vi "grafico2.vi"() -> ()   [LabVIEW 2013]
panel:
  in  "Dial":dbl(knob)
  out "Waveform Chart":dbl(graph)
  out "señal ampl 0,5 a -0,5":dbl(graph)
  in  "Numeric 3":i32
  out "Numeric 2":i32
  out "senal ampl a 5":dbl(graph)
  out "Numeric":dbl
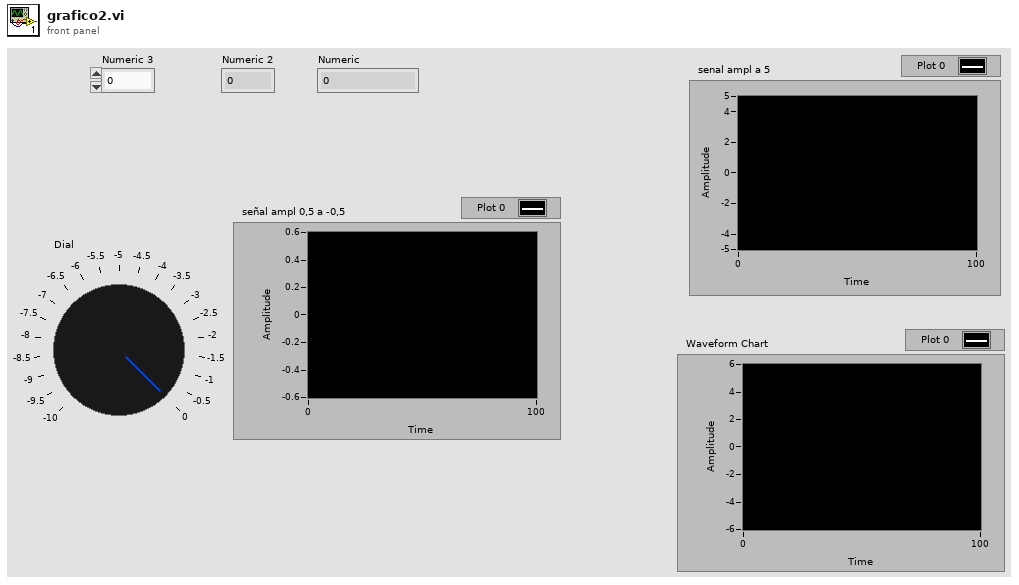
[diagram p1: front panel]
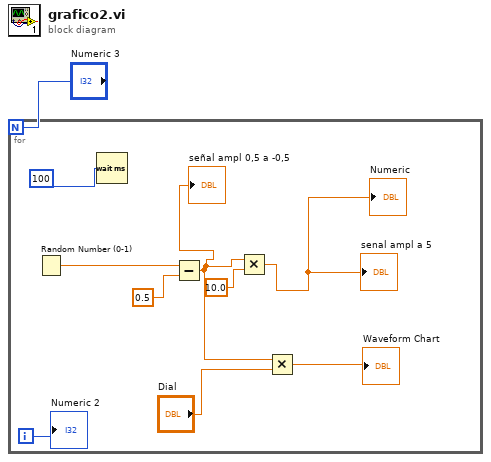
[diagram p0: block diagram]
diagram:
  n1 = for {
    N: "Numeric 3" -> [_]
    i -> [w10]
    n2 = Random Number (0-1)() -> (number: 0 to 1=w7:dbl)
    n3 = Wait (ms)(milliseconds to wait=u32 100) -> ()  [unwired: 1 out]
    n4 = Subtract(x=w7, y=0.5) -> (x-y=w4:dbl)
    "señal ampl 0,5 a -0,5" <- w4
    n5 = Multiply(x=w4, y=10.0) -> (x*y=→"Numeric" →"senal ampl a 5":dbl)
    n6 = Multiply(x=w4, y="Dial") -> (x*y=→"Waveform Chart":dbl)
    "Numeric 2" <- w10
  }
